vi "Delay.vi"(8 "Error In":errorcluster caption="错误输入", 11 "数值输入控件":u32) -> (0 "Error Out":errorcluster caption="错误输出")   [LabVIEW 2013]
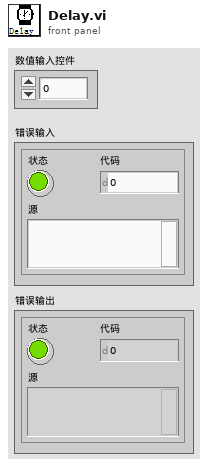
[diagram p1: front panel]
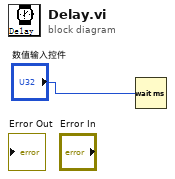
[diagram p0: block diagram]
diagram:
  n1 = Wait (ms)(milliseconds to wait="数值输入控件") -> ()  [unwired: 1 out]
